vi "Rotate Point Array.vi"(6 "Para":cluster{"Absolute?":bool, "Angle":dbl}={"Absolute?"=TRUE, "Angle"=0.0}, 8 "错误输入":errorcluster, 10 "Center":T1, 11 "Point Array":T1[](array[typedef])) -> (0 "错误输出":errorcluster, 2 "Rotated Relative Point Array":T1[](array[typedef]), 3 "Rotated Absolute Point Array":T1[](array[typedef]))   [LabVIEW 2012, in "Picture Box Tools.lvlib" / "Basic Shape.lvlib"]
uses:
  Basic Shape.lvlib
  Point Custom Control.ctl
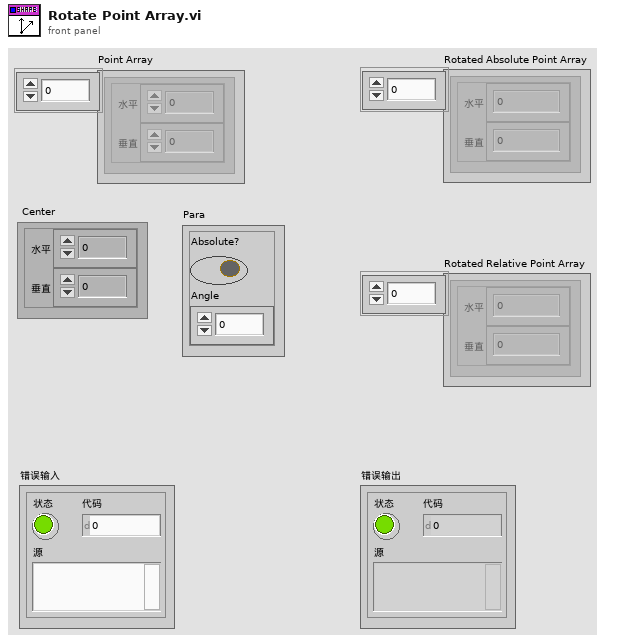
[diagram p1: front panel]
types:
  T1 = typedef "Picture Box Tools.lvlib/Basic Shape.lvlib/Point Custom Control.ctl" = cluster{"horizontal":i16, "vertical":i16}
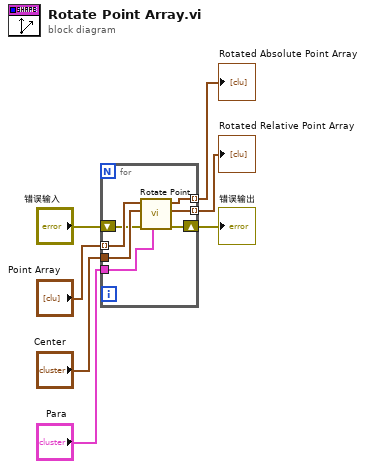
[diagram p0: block diagram]
diagram:
  n1 = for {
    tunnel: "Point Array" -> [w14] mode=indexing
    tunnel: "Center" -> [w13]
    tunnel: "Para" -> [w12]
    shift-right: [w10] -> w3
    shift-left: "错误输入" -> [w11]
    tunnel: [w9] -> w2 mode=indexing
    tunnel: [w8] -> w1 mode=indexing
    n2 = call "Rotate Point.vi"("Para"=w12, "错误输入"=w11, "Center"=w13, "Input Point"=w14) -> ("错误输出"=w10:errorcluster, "Rotated Relative Point"=w8:T1, "Rotated Absolute Point"=w9:T1)  [unwired: 5 in]
  }
  "错误输出" <- w3
  "Rotated Absolute Point Array" <- w2
  "Rotated Relative Point Array" <- w1
